vi "GetState.vi"(8 "error in (no error)":errorcluster, 11 "ControlState in":T1 {"ChainMask" format="0x%02x"}) -> (0 "error out":errorcluster, 2 "State":string, 3 "ControlState out":T1 {"ChainMask" format="0x%02x"})   [LabVIEW 2020, in "ArduinoSerialBling.lvlib"]
uses:
  ArduinoSerialBling.lvlib
  ControlState.ctl
  ChainState.ctl
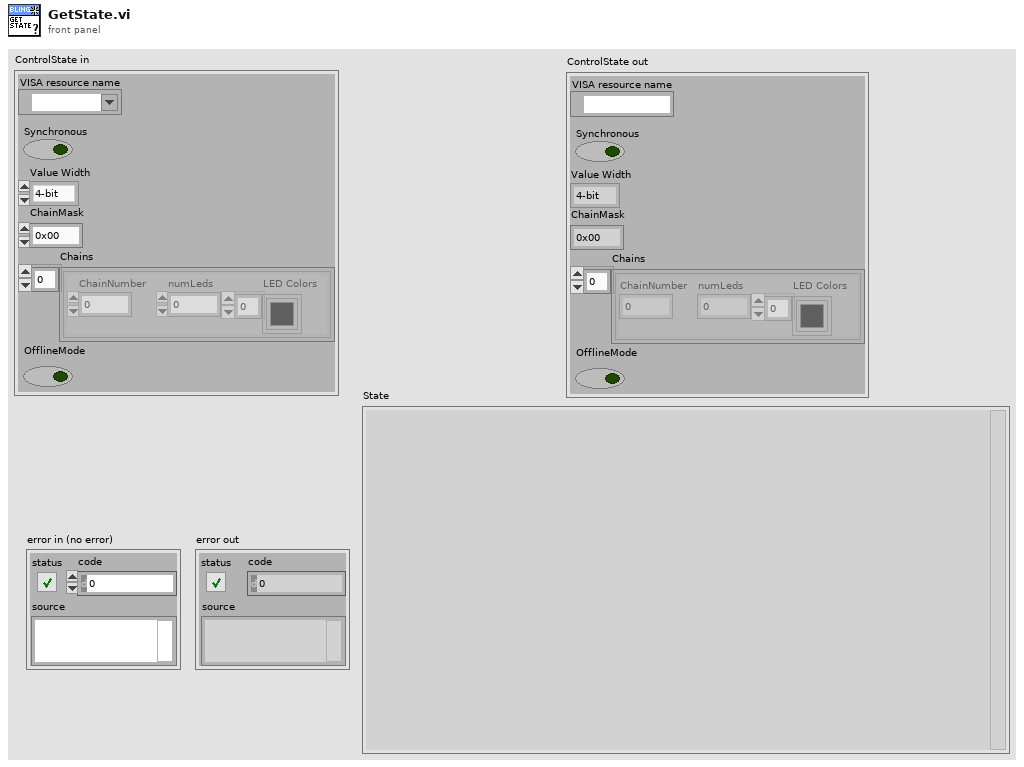
[diagram p1: front panel]
types:
  T1 = typedef "ArduinoSerialBling.lvlib/ControlState.ctl" = cluster{"VISA resource name":refnum<visa-resource-name>, "Synchronous":bool, "Value Width":enum16{"4-bit", "8-bit"}, "ChainMask":u8, "Chains":T2[], "OfflineMode":bool}
  T2 = typedef "ArduinoSerialBling.lvlib/ChainState.ctl" = cluster{"ChainNumber":u8, "numLeds":u8, "LED Colors":u32[]}
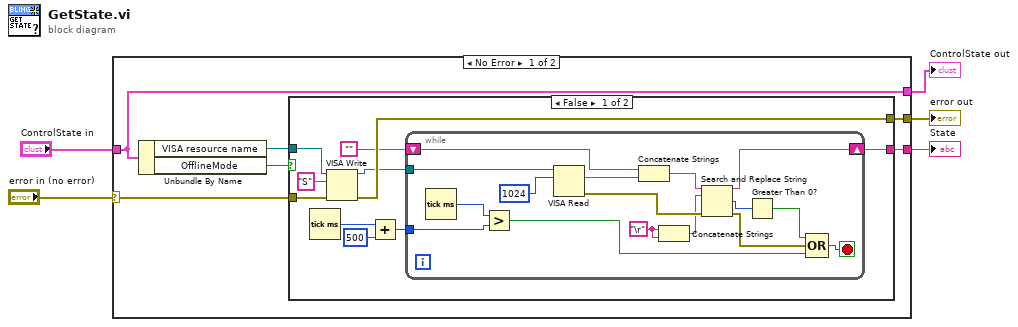
[diagram p0: block diagram]
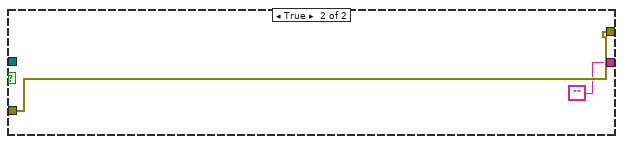
[diagram p2: hidden frame]
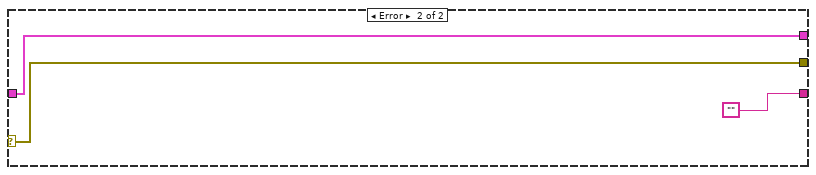
[diagram p3: hidden frame]
diagram:
  n1 = case shown="No Error" "error in (no error)" {
    selector: "error in (no error)" -> [w11 w41]
    tunnel: "ControlState in" -> [w9 w42]
    tunnel: [w7 ""] -> w3
    tunnel: [w8 w41] -> w2
    tunnel: [w9 w42] -> w1
    frame No Error {
      n2 = Unbundle By Name(w9) -> ("VISA resource name"=w10:refnum<visa-resource-name>, "OfflineMode"=w6:bool)
      n3 = case shown="False" w6 {
        tunnel: w11 -> [w21 w39]
        tunnel: w10 -> [w19 _]
        tunnel: [w18 w39] -> w8
        tunnel: [w15 ""] -> w7
        frame False {
          n4 = Tick Count (ms)() -> (millisecond timer value=w14:u32)
          n5 = VISA Write(VISA resource name=w19, write buffer="S", error in (no error)=w21) -> (VISA resource name out=w17:refnum<visa-resource-name>, error out=w18:errorcluster)  [unwired: 1 out]
          n6 = Add(x=w14, y=u32 500) -> (x+y=w13:u32)
          n7 = while {
            tunnel: w17 -> [w36]
            shift-right: [w31] -> w15
            shift-left: "" -> [w34]
            tunnel: w13 -> [w29]
            stop <- w28 stop-if-true
            w22 = "\r"
            n8 = Tick Count (ms)() -> (millisecond timer value=w30:u32)
            n9 = Greater?(x=w30, y=w29) -> (0:w27:bool)
            n10 = VISA Read(VISA resource name=w36, byte count=u32 1024) -> (read buffer=w35:string, error out=w26:errorcluster)  [unwired: 1 in, 2 out]
            n11 = Concatenate Strings(w34, w35) -> (w32:string)
            n12 = Concatenate Strings(w22, w22) -> (w23:string)
            n13 = Search and Replace String(input string=w32, search string=w23, error in=w26) -> (result string=w31:string, number of replacements=w33:i32, error out=w24:errorcluster)  [unwired: 5 in, 1 out]
            n14 = Greater Than 0?(x=w33) -> (x > 0?=w25:bool)
            n15 = Compound Arithmetic op=OR(w25, w24, w27) -> (w28:bool)
          }
        }
        frame True {
        }
      }
    }
    frame Error {
    }
  }
  "ControlState out" <- w1
  "error out" <- w2
  "State" <- w3
